vi "Init Device.vi"(8 "error in (no error)":errorcluster, 11 "Synchronization Device in":refnum<class "NI DAQ.lvclass">) -> (0 "error out":errorcluster, 3 "Synchronization Device out":refnum<class "NI DAQ.lvclass">)   [LabVIEW 2023, in "NI DAQ.lvlib" / "NI DAQ.lvclass"]
uses:
  NI DAQ.lvclass
  Sync Device/Sync Device.lvclass
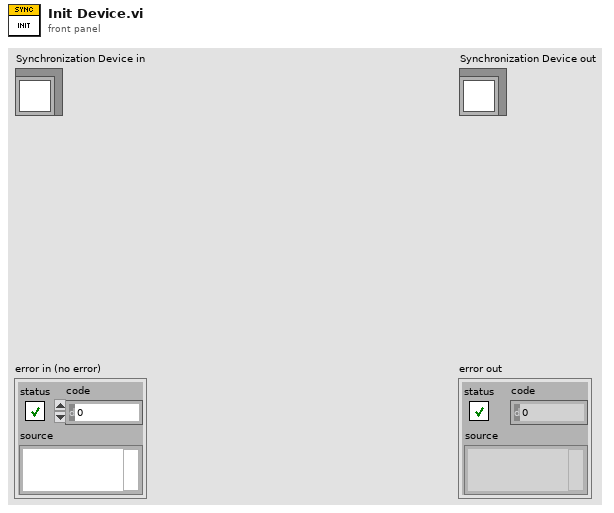
[diagram p1: front panel]
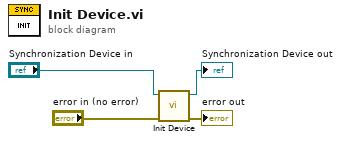
[diagram p0: block diagram]
diagram:
  n1 = call-parent "Init Device.vi"("error in (no error)"="error in (no error)", "Device in"="Synchronization Device in") -> ("error out"=→"error out":errorcluster, "Device out"=→"Synchronization Device out":refnum<class "NI DAQ.lvclass">)  [unwired: 8 in]
